vi "toDate.vi"(8 "error in (no error)":errorcluster, 11 "Variant":variant) -> (0 "error out":errorcluster, 3 "time stamp":timestamp)   [LabVIEW 2018, in "Account History.lvclass"]
uses:
  Account History.lvclass
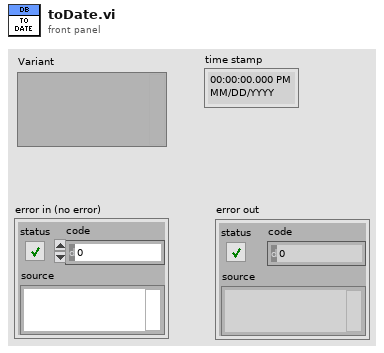
[diagram p1: front panel]
types:
  T1 = typedef "LVDateTimeRec.ctl" = cluster{"fractional second":dbl, "second":i32, "minute":i32, "hour":i32, "day of month":i32, "month":i32, "year":i32, "day of week":i32, "day of year":i32, "DST":i32}
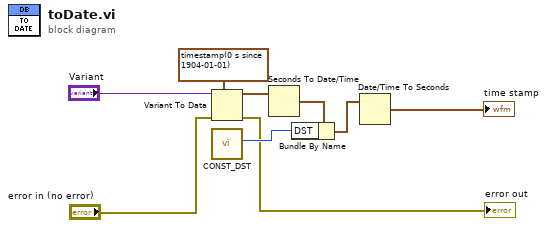
[diagram p0: block diagram]
diagram:
  n1 = Variant To Data(error in="error in (no error)", type=timestamp(0 s since 1904-01-01), Variant="Variant") -> (data=w6:timestamp, error out=→"error out":errorcluster)
  n2 = call "CONST_DST.vi"() -> ("DST"=w9:i32)  [unwired: 11 in]
  n3 = Seconds To Date/Time(time stamp (now)=w6) -> (date time rec=w7:T1)  [unwired: 1 in]
  n4 = Bundle By Name(cluster=w7, "DST"=w9) -> (w8:T1)
  n5 = Date/Time To Seconds(2:w8) -> (0:→"time stamp":timestamp)  [unwired: 1 in]
